vi "arduino_subVi.vi"(2 "Command 2":string="led_on", 3 "VISA resource name 2":refnum<visa-resource-name>) -> (0 "Commentary 2":string, 1 "VISA resource name out":refnum<visa-resource-name>)   [LabVIEW 2018]
uses:
  <vilib>/Instr/_visa.llb/VISA Configure Serial Port (Instr).vi
panel:
  out "return count":u32
  out "error out":errorcluster
  # "D2_on\nD2_off\nled_on\nled_off"
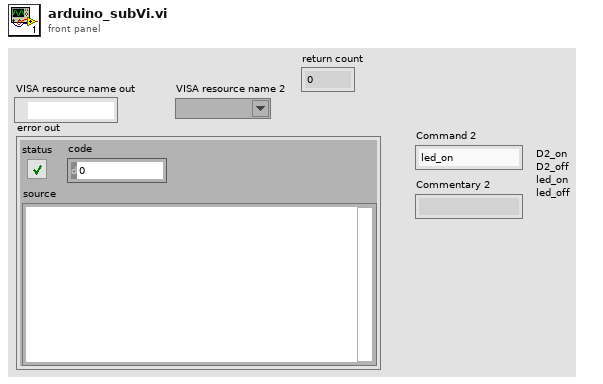
[diagram p1: front panel]
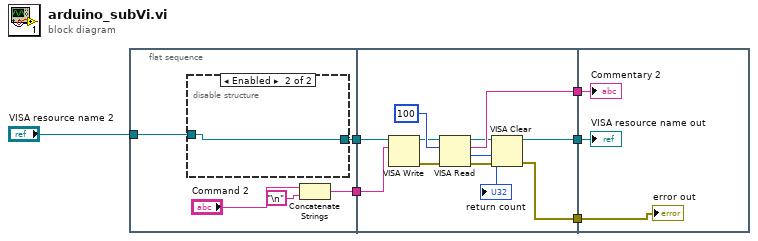
[diagram p0: block diagram]
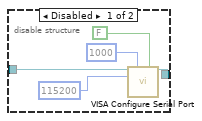
[diagram p2: hidden frame]
diagram:
  n1 = flat-sequence {
    tunnel: [w11] -> w5
    tunnel: [w8] -> w2
    tunnel: "VISA resource name 2" -> [w7]
    tunnel: [w25] -> w6
    tunnel: w5 -> [w27]
    tunnel: [w28] -> w4
    tunnel: [w23] -> w3
    tunnel: w2 -> [w21]
    tunnel: w6 -> [w30]
    tunnel: w4 -> [w31]
    tunnel: w3 -> [w29]
    frame #0 {
      n2 = disable-structure shown="Enabled" {
        disable-tunnel: [w16 w17] -> w11
        disable-tunnel: w7 -> [w12 w17]
        frame Disabled {
          n3 = call-poly "VISA Configure Serial Port"("VISA resource name"=w12, "timeout (10sec)"=u32 1000, "Enable Termination\nChar (T)"=FALSE ("Enable Termination\nChar (T)"), "baud rate (9600)"=u32 115200) -> ("VISA resource name out"=w16:refnum<visa-resource-name>)  [unwired: 10 in, 1 out]
        }
        frame Enabled {
        }
      }
      n4 = Concatenate Strings("Command 2", "\n") -> (w8:string)
    }
    frame #1 {
      n5 = VISA Write(VISA resource name=w27, write buffer=w21) -> (VISA resource name out=w20:refnum<visa-resource-name>, error out=w19:errorcluster)  [unwired: 1 in, 1 out]
      n6 = VISA Read(VISA resource name=w20, byte count=u32 100, error in (no error)=w19) -> (VISA resource name out=w26:refnum<visa-resource-name>, read buffer=w28:string, return count=→"return count":u32, error out=w24:errorcluster)
      n7 = VISA Clear(VISA resource name=w26, error in (no error)=w24) -> (VISA resource name out=w25:refnum<visa-resource-name>, error out=w23:errorcluster)
    }
    frame #2 {
      "Commentary 2" <- w31
      "VISA resource name out" <- w30
      "error out" <- w29
    }
  }
